vi "Motion Profile Generator-Demo.vi"(0 "Max Speed (rotations/sec)":dbl=3.0, 5 "Max Acceleration (rotations/sec^2)":dbl=1.0, 7 "Max Jerk (rotations/sec^3)":dbl=1.0, 9 "Rotations to Travel":dbl=4.0, 11 "Motion Profile Control Frame Rate":dbl=10.0) -> (4 "Position rotations":dbl[](array[numeric]), 6 "velocity rotations/sec":dbl[](array[numeric]), 8 "acceleration rotations/sec^2":dbl[](array[numeric]), 10 "XY Graph":cluster{dbl[], dbl[]}[](graph))   [LabVIEW 2015]
panel:
  out "Final Position":dbl
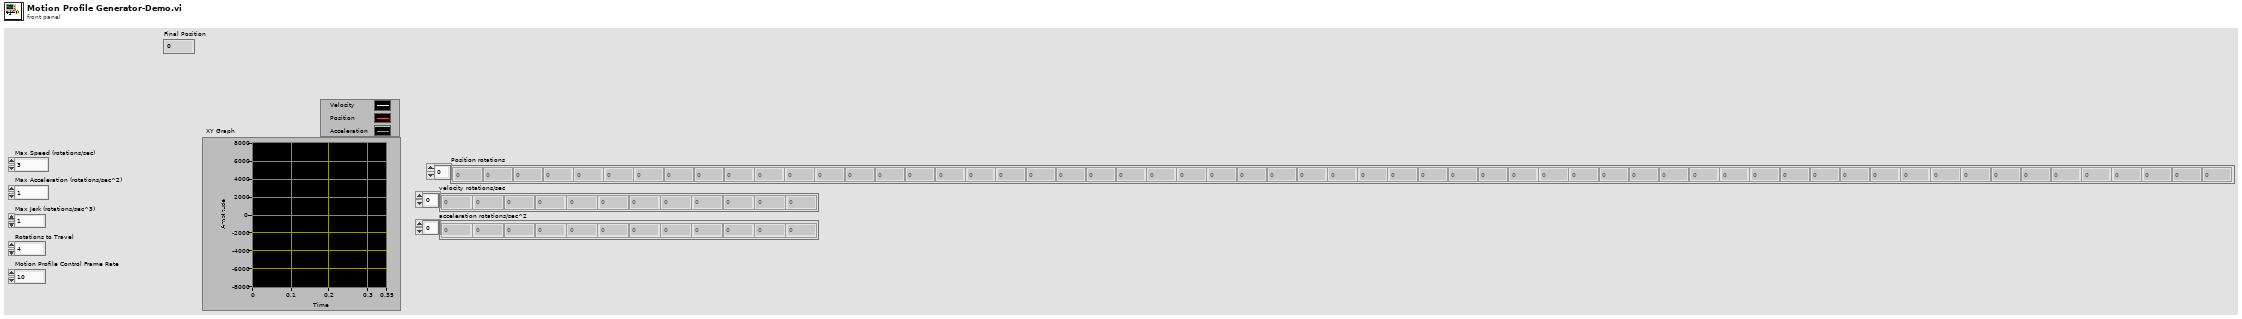
[diagram p1: front panel]
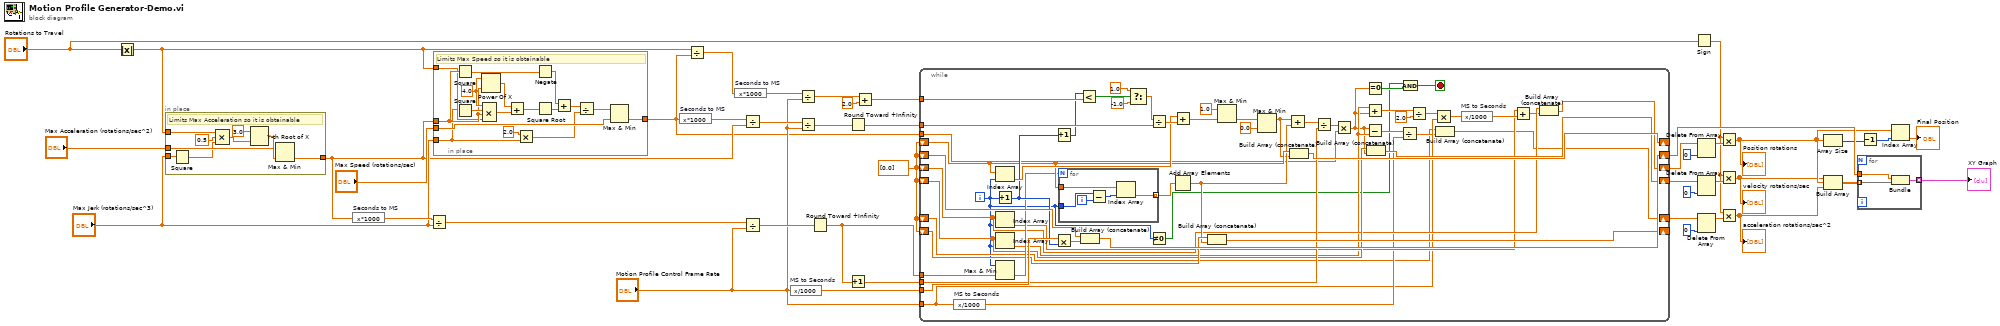
[diagram p0: block diagram]
diagram:
  w27 = dbl[] [0.0]
  n1 = Absolute Value(x="Rotations to Travel") -> (abs(x)=w6:dbl)
  n2 = in-place {
    in-place-border: "Max Jerk (rotations/sec^3)" -> [w52]
    in-place-border: "Max Acceleration (rotations/sec^2)" -> [w50]
    in-place-border: [w49] -> w17
    in-place-border: w6 -> [w48]
    # "Limits Max Acceleration so it is obtainable"
    n3 = Square(x=w52) -> (x^2=w46:dbl)
    n4 = Compound Arithmetic op=MULTIPLY(w48, 0.5 ("value"), w46) -> (w45:dbl)
    n5 = Y-th Root of X(1:w45, 2:3.0 ("y")) -> (0:w51:dbl)
    n6 = Max & Min(x=w50, y=w51) -> (min(x,y)=w49:dbl)  [unwired: 1 out]
  }
  n7 = expression code="x*1000" "Seconds to MS"(w17) -> (w42:dbl)
  n8 = Divide(x=w42, y="Max Jerk (rotations/sec^3)") -> (x/y=w32:dbl)
  n9 = in-place {
    in-place-border: "Max Speed (rotations/sec)" -> [w69]
    in-place-border: [w56] -> w16
    in-place-border: w17 -> [w62]
    in-place-border: w6 -> [w61]
    in-place-border: "Max Jerk (rotations/sec^3)" -> [w58]
    w65 = 4.0 ("x")
    # "Limits Max Speed so it is obtainable"
    n10 = Square(x=w62) -> (x^2=w68:dbl)
    n11 = Square(x=w58) -> (x^2=w64:dbl)
    n12 = Power Of X(1:w62, 2:w65) -> (0:w66:dbl)
    n13 = Compound Arithmetic op=MULTIPLY(w65, w64, w62, w61) -> (w63:dbl)
    n14 = Add(x=w66, y=w63) -> (x+y=w60:dbl)
    n15 = Multiply(x=2.0, y=w58) -> (x*y=w53:dbl)
    n16 = Negate(x=w68) -> (-x=w67:dbl)
    n17 = Square Root(x=w60) -> (sqrt(x)=w57:dbl)
    n18 = Add(x=w67, y=w57) -> (x+y=w55:dbl)
    n19 = Divide(x=w55, y=w53) -> (x/y=w54:dbl)
    n20 = Max & Min(x=w54, y=w69) -> (min(x,y)=w56:dbl)  [unwired: 1 out]
  }
  n21 = expression code="x*1000" "Seconds to MS"(w16) -> (w41:dbl)
  n22 = Divide(x=w6, y=w16) -> (x/y=w40:dbl)
  n23 = expression code="x*1000" "Seconds to MS"(w40) -> (w39:dbl)
  n24 = Divide(x=w41, y=w17) -> (x/y=w35:dbl)
  n25 = Divide(x=w32, y="Motion Profile Control Frame Rate") -> (x/y=w31:dbl)
  n26 = expression code="x/1000" "MS to Seconds"("Motion Profile Control Frame Rate") -> (w43:dbl)
  n27 = Divide(x=w39, y="Motion Profile Control Frame Rate") -> (x/y=w38:dbl)
  n28 = Divide(x=w35, y="Motion Profile Control Frame Rate") -> (x/y=w34:dbl)
  n29 = Round Toward +Infinity(x=w31) -> (ceil(x): smallest int >= x=w30:dbl)
  n30 = Round Toward +Infinity(x=w34) -> (ceil(x): smallest int >= x=w33:dbl)
  n31 = Increment(x=w30) -> (x+1=w29:dbl)
  n32 = Add(x=w38, y=2.0) -> (x+y=w36:dbl)
  n33 = while {
    shift-right: [w122] -> w25
    shift-left: w27 -> [w123]
    tunnel: w43 -> [w121]
    tunnel: w36 -> [w119]
    shift-right: [w105] -> _
    shift-left: w27 -> [w104]
    tunnel: w33 -> [w111]
    tunnel: w30 -> [w102]
    shift-right: [w99] -> _
    shift-left: w27 -> [w100]
    tunnel: w29 -> [w95]
    tunnel: w16 -> [w93]
    shift-right: [w92] -> w11
    shift-left: w27 -> [w90]
    shift-right: [w91] -> w9
    shift-left: w27 -> [w84]
    tunnel: "Motion Profile Control Frame Rate" -> [w78]
    shift-right: [w76] -> w13
    shift-left: w27 -> [w75]
    i -> [w74]
    stop <- w70 stop-if-true
    n34 = expression code="x/1000" "MS to Seconds"(w78) -> (w79:dbl)
    n35 = Index Array(array=w104, index=w74) -> (element=w109:dbl)
    n36 = Increment(x=w74) -> (x+1=w107:i32)
    n37 = Index Array(array=w84, index=w74) -> (element=w83:dbl)
    n38 = Index Array(array=w90, index=w74) -> (element=w81:dbl)
    n39 = Max & Min(x=w74, y=w102) -> (min(x,y)=w101:dbl)  [unwired: 1 out]
    n40 = Increment(x=w107) -> (x+1=w108:i32)
    n41 = Multiply(x=w121, y=w107) -> (x*y=w120:dbl)
    n42 = for {
      N: w101 -> [_]
      tunnel: w74 -> [w127]
      tunnel: w104 -> [w125]
      tunnel: [w124] -> w103 mode=indexing
      i -> [w128]
      n43 = Subtract(x=w127, y=w128) -> (x-y=w126:i32)
      n44 = Index Array(array=w125, index=w126) -> (element=w124:dbl)
    }
    n45 = Less?(x=w108, y=w119) -> (x < y?=w115:bool)
    n46 = Build Array (concatenate)(w123, w120) -> (w122:dbl[])
    n47 = Select(t=1.0, s=w115, f=-1.0) -> (s? t:f=w112:dbl)
    n48 = Divide(x=w112, y=w111) -> (x/y=w110:dbl)
    n49 = Not Equal To 0?(x=w74) -> (x != 0?=w71:bool)
    n50 = Add(x=w109, y=w110) -> (x+y=w106:dbl)
    n51 = Add Array Elements(numeric array=w103) -> (sum=w98:dbl)
    n52 = Build Array (concatenate)(w100, w98) -> (w99:dbl[])
    n53 = Max & Min(x=1.0, y=w106) -> (min(x,y)=w117:dbl)  [unwired: 1 out]
    n54 = Max & Min(x=w117, y=0.0) -> (max(x,y)=w97:dbl)  [unwired: 1 out]
    n55 = Add(x=w97, y=w98) -> (x+y=w96:dbl)
    n56 = Build Array (concatenate)(w104, w97) -> (w105:dbl[])
    n57 = Divide(x=w96, y=w95) -> (x/y=w94:dbl)
    n58 = Multiply(x=w94, y=w93) -> (x*y=w73:dbl)
    n59 = Add(x=w81, y=w73) -> (x+y=w89:dbl)
    n60 = Subtract(x=w73, y=w81) -> (x-y=w80:dbl)
    n61 = Equal To 0?(x=w73) -> (x = 0?=w72:bool)
    n62 = Build Array (concatenate)(w90, w73) -> (w92:dbl[])
    n63 = Divide(x=w80, y=w79) -> (x/y=w77:dbl)
    n64 = And(x=w71, y=w72) -> (x .and. y?=w70:bool)
    n65 = Divide(x=w89, y=2.0) -> (x/y=w87:dbl)
    n66 = Multiply(x=w87, y=w78) -> (x*y=w86:dbl)
    n67 = Build Array (concatenate)(w75, w77) -> (w76:dbl[])
    n68 = expression code="x/1000" "MS to Seconds"(w86) -> (w85:dbl)
    n69 = Add(x=w83, y=w85) -> (x+y=w82:dbl)
    n70 = Build Array (concatenate)(w84, w82) -> (w91:dbl[])
  }
  n71 = Sign(1:"Rotations to Travel") -> (0:w1:dbl)
  n72 = Delete From Array(array=w9, index=0) -> (array with subset deleted=w8:dbl[])  [unwired: 1 in, 1 out]
  n73 = Delete From Array(array=w11, index=0) -> (array with subset deleted=w7:dbl[])  [unwired: 1 in, 1 out]
  n74 = Delete From Array(array=w13, index=0) -> (array with subset deleted=w12:dbl[])  [unwired: 1 in, 1 out]
  n75 = Multiply(x=w1, y=w8) -> (x*y=w4:dbl[])
  "Position rotations" <- w4
  n76 = Multiply(x=w1, y=w7) -> (x*y=w3:dbl[])
  "velocity rotations/sec" <- w3
  n77 = Multiply(x=w1, y=w12) -> (x*y=w2:dbl[])
  "acceleration rotations/sec^2" <- w2
  n78 = Array Size(array=w4) -> (size(s)=w23:i32)
  n79 = Build Array(w3, w4, w2) -> (w26:dbl[][])
  n80 = for {
    tunnel: w26 -> [w131] mode=indexing
    tunnel: w25 -> [w130]
    tunnel: [w129] -> w24 mode=indexing
    n81 = Bundle(w130, w131) -> (w129:cluster{dbl[], dbl[]})  [unwired: 1 in]
  }
  "XY Graph" <- w24
  n82 = Decrement(x=w23) -> (x-1=w22:i32)
  n83 = Index Array(array=w4, index=w22) -> (element=→"Final Position":dbl)
